vi "Engine UI Msg Callback.vi"(4 "User Parameter":variant, 5 "Event Data":cluster{"msg":refnum<k7>}, 6 "Control Ref":refnum<k7>, 7 "Event Common Data":T2) -> ()   [LabVIEW 2020, in "TSS.lvlib" / "Engine.lvclass"]
uses:
  Engine.lvclass
  Data Types/UIMsg.ctl
  Engine.lvclass/Engine.ctl
  UIMessage/UIMessage.lvclass
  TSS.lvlib
panel:
  out "UIMsg":T1
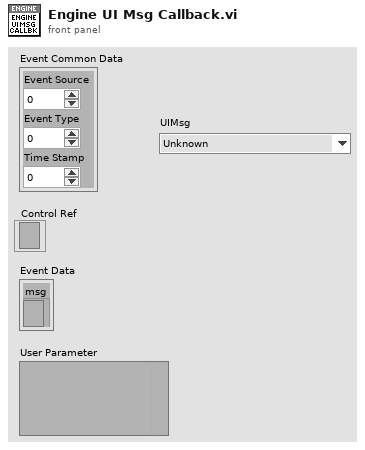
[diagram p1: front panel]
types:
  T1 = typedef "TSS.lvlib/UIMsg.ctl" = enum16{"Unknown", "BreakOnUserRequest", "BreakOnBreakpoint", "BreakOnRunTimeError", "Trace", "TerminatingExecution", "AbortingExecution", "KillingExecutionThreads", "EndExecution", "ShutDownComplete", "StartExecution", "ProgressPercent", "ProgressText", "StartInteractiveExecution", "EndInteractiveExecution", "TerminatingInteractiveExecution", "TerminationCancelled", "ResumeFromBreak", "StartFileExecution", "EndFileExecution", "ShutDownCancelled", "LocalizationSettingChanged", "OpenWindows", "TileWindows", "CascadeWindows", "ReportChanged", "CloseWindows", "RefreshWindows", "ClientFileChanged", "DisplayReport", "ModelState_Initializing", "ModelState_Waiting", "ModelState_Identified", "ModelState_BeginTesting", "ModelState_TestingComplete", "ModelState_PostProcessingComplete", "ModelState_EnabledStateSet", "ReportLocationChanged", "GotoLocation", "PushUndoItem", "OutputMessages", "TypePaletteFileListChanged", "NonTerminatingThreadsArePreventingTermination", "ModelState_PostProcessing", "ReportCollectionChanged", "RuntimeError"}
  T2 = cluster{"Event Source":i32, "Event Type":u32, "Time Stamp":u32}
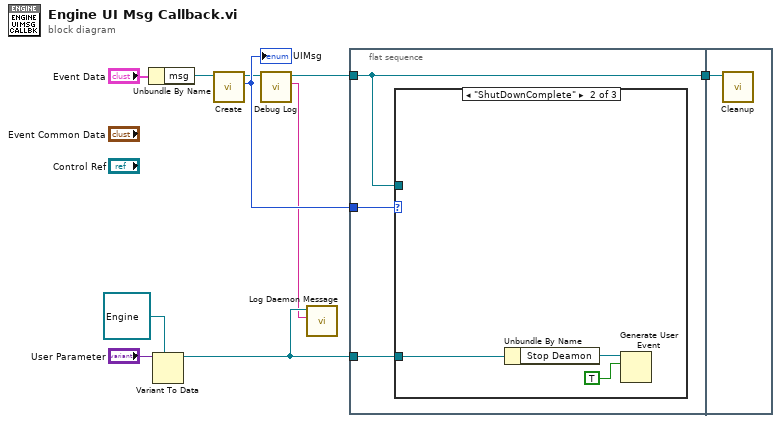
[diagram p0: block diagram]
diagram:
  n1 = Unbundle By Name("Event Data") -> ("msg"=w6:refnum<k7>)
  n2 = Variant To Data(type=refnum<class "Engine.lvclass"> refnum ("TSEngine"), Variant="User Parameter") -> (data=w7:refnum<class "Engine.lvclass">)  [unwired: 1 in, 1 out]
  n3 = call "Create.vi"("msg"=w6) -> ("Code"=w5:T1, "UIMessage out"=w3:refnum<class "UIMessage.lvclass">)  [unwired: 8 in, 1 out]
  "UIMsg" <- w5
  n4 = call "Debug Log.vi"("UIMessage in"=w3) -> ("Debug Line"=w1:string, "UIMessage out"=w2:refnum<class "UIMessage.lvclass">)  [unwired: 8 in, 1 out]
  n5 = call "Log Daemon Message.vi"("Line"=w1, "Engine in"=w7) -> ()  [unwired: 8 in, 2 out]
  n6 = flat-sequence {
    tunnel: w7 -> [w13]
    tunnel: w5 -> [w12]
    tunnel: w2 -> [w11]
    tunnel: [w11] -> w4
    tunnel: w4 -> [w17]
    frame #0 {
      n7 = case shown="\"ShutDownComplete\"" w12 {
        tunnel: w13 -> [_ w16 _]
        tunnel: w11 -> [_ _ _]
        frame Default {
        }
        frame "ShutDownComplete" {
          # "Can finish shutting down"
          n8 = Unbundle By Name(w16) -> ("Stop Deamon"=w15:refnum<user-event>)
          n9 = Generate User Event(user event=w15, event data cluster=TRUE ("event data")) -> ()  [unwired: 2 in, 2 out]
        }
        frame "ShutDownCancelled" {
        }
      }
    }
    frame #1 {
      n10 = call "Cleanup.vi"("UIMessage in"=w17) -> ()  [unwired: 10 in, 1 out]
    }
  }
